vi "合法项目集合.vi"() -> ()   [LabVIEW 2013]
panel:
  in  "合法项目集合":string[](array[string])=["168", "196", "DR96", "195"]
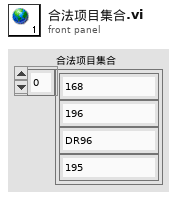
[diagram p1: front panel]
diagram:
